vi "In_ON.vi"(8 "error in":errorcluster, 9 "Protocol parameters":T2={"Repetitions"=1.0, "ON time"=40.0, "OFF time"=120.0, "Stim onset"=5.0, "Stim frequency"=1.0, "Pulse width"=1.0, "Acquire before ON"=1.0, "Acquire after ON"=1.0, "Sync shutter to acquisition"=TRUE} {"Pulse width" min=0.0001 max=0.1 step=0.01; "Acquire after ON" min=0.0 max=10.0 step=1.0; "Acquire before ON" min=0.0 max=10.0 step=1.0; "Repetitions" min=1.0 max=10.0 step=1.0; "OFF time" min=0.0 max=1000.0; "ON time" min=0.0 max=1000.0; "Stim onset" min=0.0 max=100.0; "Stim frequency" min=0.1 max=40.0 step=1.0}, 10 "Device parameters":T3={"Triggered?"=FALSE, "Shutter channel"="", "Acquisition channels"="", "Acquisition sample rate"=100.0, "Read chunk size"=0, "Stimulation channel"="Dev1/ao0", "Stimulation sample rate"=100.0} {"Read chunk size" min=100 max=100000; "Acquisition sample rate" min=10.0 max=10000.0 step=10.0; "Stimulation sample rate" min=10.0 max=10000.0}, 11 "Read position":i32) -> (0 "error out":errorcluster, 1 "Finished?":bool, 2 "Do acquire":bool, 3 "Where":T1)   [LabVIEW 2010]
uses:
  typedefs/device_parameters.ctl
  typedefs/protocol_parameters.ctl
  typedefs/where_in_protocol_cluster.ctl
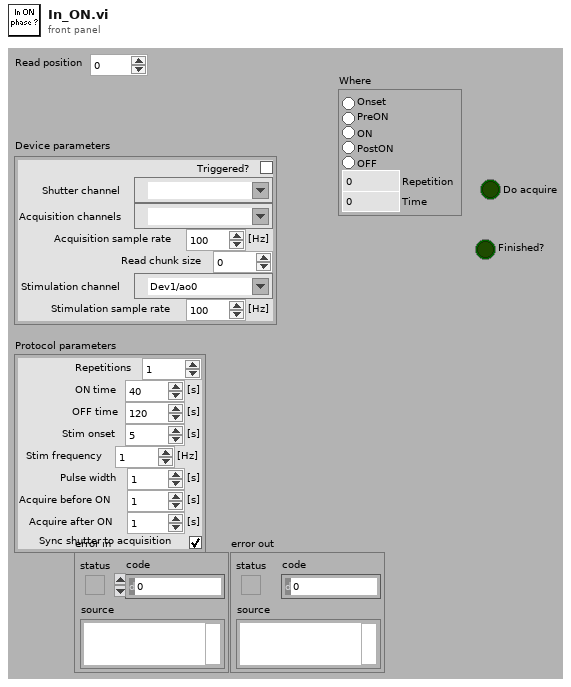
[diagram p1: front panel]
types:
  T1 = typedef "where_in_protocol_cluster.ctl" = cluster{"Onset":bool, "PreON":bool, "ON":bool, "PostON":bool, "OFF":bool, "Repetition":dbl, "Time":dbl}
  T2 = typedef "protocol_parameters.ctl" = cluster{"Repetitions":dbl, "ON time":dbl, "OFF time":dbl, "Stim onset":dbl, "Stim frequency":dbl, "Pulse width":dbl, "Acquire before ON":dbl, "Acquire after ON":dbl, "Sync shutter to acquisition":bool}
  T3 = typedef "device_parameters.ctl" = cluster{"Triggered?":bool, "Shutter channel":tag, "Acquisition channels":tag, "Acquisition sample rate":dbl, "Read chunk size":i32, "Stimulation channel":tag, "Stimulation sample rate":dbl}
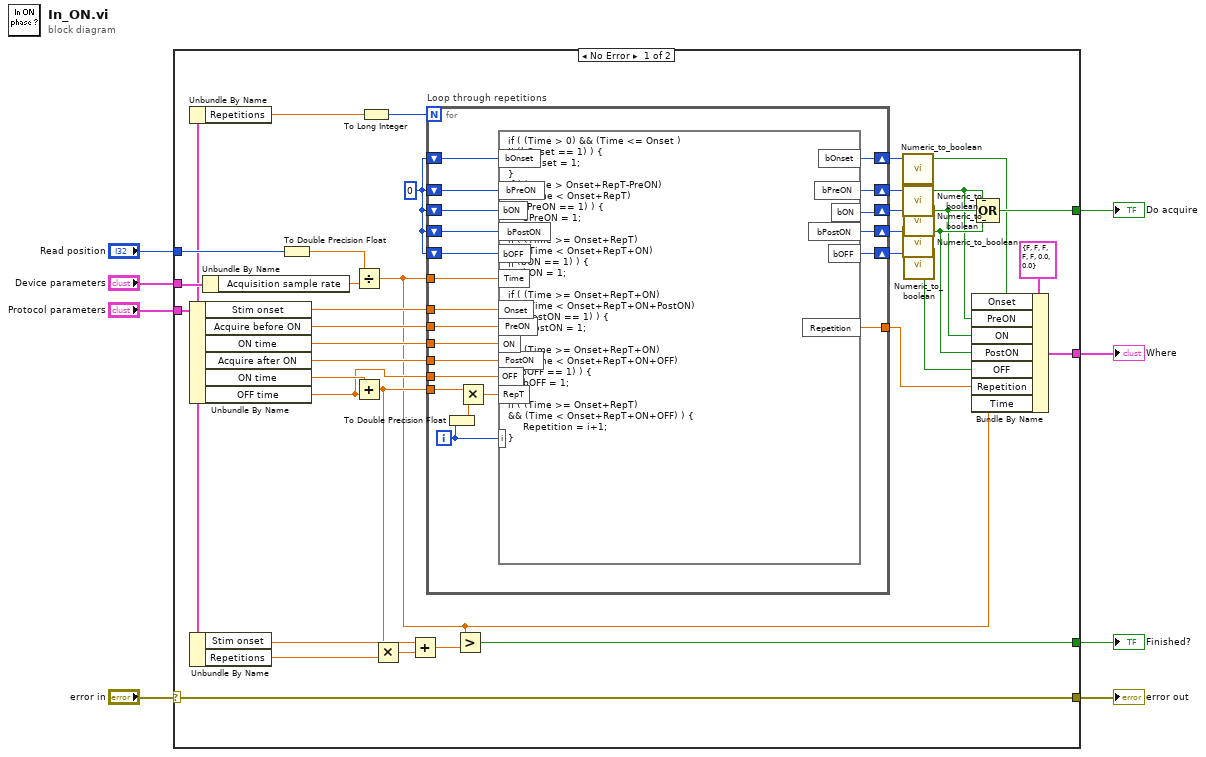
[diagram p0: block diagram]
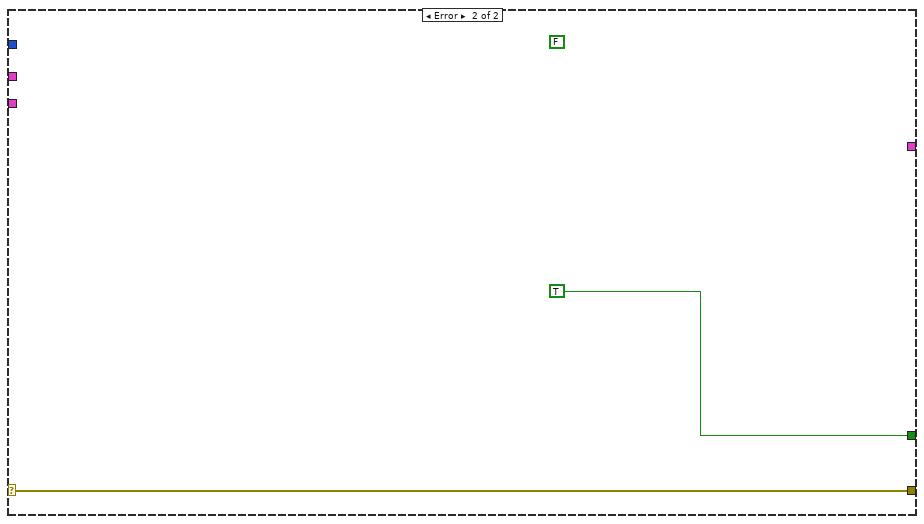
[diagram p2: hidden frame]
diagram:
  n1 = case shown="No Error" "error in" {
    selector: "error in" -> [w44 w67]
    tunnel: [w44 w67] -> w7
    tunnel: "Device parameters" -> [w43 _]
    tunnel: "Protocol parameters" -> [w36 _]
    tunnel: "Read position" -> [w38 _]
    tunnel: [w31 TRUE] -> w3
    tunnel: [w22 _] -> w2
    tunnel: [w17 _] -> w1
    frame No Error {
      w19 = 0
      n2 = Unbundle By Name(w36) -> ("Repetitions"=w40:dbl)
      n3 = Unbundle By Name(w36) -> ("Stim onset"=w30:dbl, "Acquire before ON"=w29:dbl, "ON time"=w28:dbl, "Acquire after ON"=w27:dbl, "ON time"=w41:dbl, "OFF time"=w21:dbl)
      n4 = Unbundle By Name(w36) -> ("Stim onset"=w33:dbl, "Repetitions"=w35:dbl)
      n5 = Unbundle By Name(w43) -> ("Acquisition sample rate"=w42:dbl)
      n6 = To Double Precision Float(number=w38) -> (double precision float=w37:dbl)
      n7 = Divide(x=w37, y=w42) -> (x/y=w15:dbl)
      n8 = Add(x=w41, y=w21) -> (x+y=w26:dbl)
      n9 = To Long Integer(number=w40) -> (32bit integer=w39:i32)
      n10 = Multiply(x=w26, y=w35) -> (x*y=w34:dbl)
      n11 = Add(x=w33, y=w34) -> (x+y=w32:dbl)
      n12 = for "Loop through repetitions" {
        N: w39 -> [_]
        shift-right: [w54] -> w25
        shift-left: w19 -> [w55]
        tunnel: w15 -> [w58]
        tunnel: w29 -> [w60]
        tunnel: w30 -> [w59]
        shift-right: [w53] -> w24
        shift-left: w19 -> [w57]
        tunnel: w28 -> [w61]
        tunnel: w27 -> [w62]
        tunnel: w26 -> [w64]
        shift-right: [w52] -> w23
        shift-left: w19 -> [w56]
        shift-right: [w49] -> w20
        shift-left: w19 -> [w51]
        tunnel: w21 -> [w50]
        tunnel: [w48] -> w14
        shift-right: [w45] -> w18
        shift-left: w19 -> [w46]
        i -> [w47]
        n13 = To Double Precision Float(number=w47) -> (double precision float=w65:dbl)
        n14 = Multiply(x=w64, y=w65) -> (x*y=w63:dbl)
        n15 = formula code="if ( (Time > 0) && (Time <= Onset ) \n|| (bOnset == 1) ) {\n     bOnset = 1;\n}\nif ( (Time > Onset+RepT-PreON)\n&& (Time < Onset+RepT)\n|| (bPreON == 1) ) {\n     bPreON = 1;\n}\nif ( (Time >= Onset+RepT)\n&& (Time < Onset+RepT+ON)\n|| (bON == 1) ) {\n     bON = 1;\n}\nif ( (Time >= Onset+RepT+ON)\n&& (Time < Onset+RepT+ON+PostON)\n|| (bPostON == 1) ) {\n     bPostON = 1;\n}\nif ( (Time >= Onset+RepT+ON)\n&& (Time < Onset+RepT+ON+OFF)\n|| (bOFF == 1) ) {\n     bOFF = 1;\n}\nif ( (Time >= Onset+RepT)\n&& (Time < Onset+RepT+ON+OFF) ) {\n     Repetition = i+1;\n}"("RepT"=w63, "PostON"=w62, "ON"=w61, "PreON"=w60, "Onset"=w59, "Time"=w58, "bPreON"=w55, "bON"=w57, "bPostON"=w56, "bOFF"=w51, "OFF"=w50, "i"=w47, "bOnset"=w46) -> ("bPreON"=w54:i32, "bON"=w53:i32, "bPostON"=w52:i32, "bOFF"=w49:i32, "Repetition"=w48:dbl, "bOnset"=w45:i32)
      }
      n16 = Greater?(x=w15, y=w32) -> (0:w31:bool)
      n17 = call "Numeric_to_boolean.vi"("Numeric"=w18) -> ("Bool"=w9:bool)  [unwired: 4 in]
      n18 = call "Numeric_to_boolean.vi"("Numeric"=w25) -> ("Bool"=w10:bool)  [unwired: 4 in]
      n19 = call "Numeric_to_boolean.vi"("Numeric"=w23) -> ("Bool"=w12:bool)  [unwired: 4 in]
      n20 = call "Numeric_to_boolean.vi"("Numeric"=w24) -> ("Bool"=w11:bool)  [unwired: 4 in]
      n21 = call "Numeric_to_boolean.vi"("Numeric"=w20) -> ("Bool"=w13:bool)  [unwired: 4 in]
      n22 = Bundle By Name(cluster=T1 {"Onset"=FALSE, "PreON"=FALSE, "ON"=FALSE, "PostON"=FALSE, "OFF"=FALSE, "Repetition"=0.0, "Time"=0.0} ("Where"), "Onset"=w9, "PreON"=w10, "ON"=w11, "PostON"=w12, "OFF"=w13, "Repetition"=w14, "Time"=w15) -> (w17:T1)
      n23 = Compound Arithmetic op=OR(w10, w11, w12) -> (w22:bool)
    }
    frame Error {
      (unwired) FALSE
    }
  }
  "Do acquire" <- w2
  "error out" <- w7
  "Finished?" <- w3
  "Where" <- w1
